vi "SeretBallExercise.vi"(1 "ROUND":dbl) -> ()   [LabVIEW 2013]
uses:
  <vilib>/NXT/Block Support/NXT_OutputPort.ctl
  <vilib>/NXT/Block Support/NXT_InputPort.ctl
  <vilib>/NXT/NXTIO Xnodes/NXTIONodeSubVIs/NXTStopMotors.vi
  <vilib>/NXT/Dual Mode Library/Sensors/EV3_Gyro_Angle.vi
  <vilib>/NXT/Dual Mode Library/Sensors/EV3_Gyro_Reset.vi
  <vilib>/NXT/Subs/LVHSConnector.ctl
  <vilib>/NXT/NXTIO Xnodes/AddressXNode/NXTIOAddress.xnode
  <vilib>/NXT/NXTIO Xnodes/NXTIOXNode/NXTIO.xnode
  <vilib>/NXT/LegoClasses/BrickReference/BrickReference.lvclass
panel:
  out "Numeric":dbl
  out "isBlack2":bool
  out "Degrees 2":sgl
  in  "stop 2":bool
  in  "stop":bool
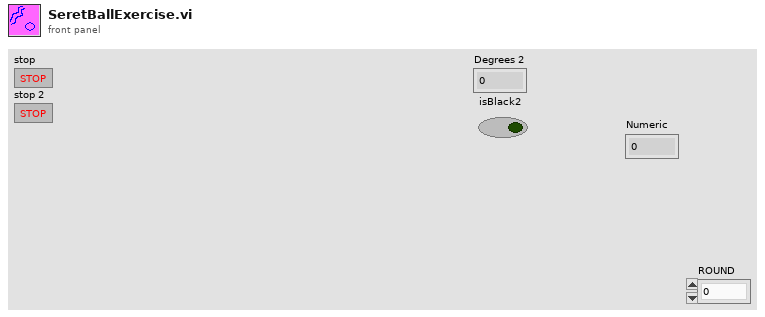
[diagram p1: front panel]
types:
  T1 = typedef "NXT_OutputPort.ctl" = u8
  T2 = typedef "NXT_InputPort.ctl" = u32
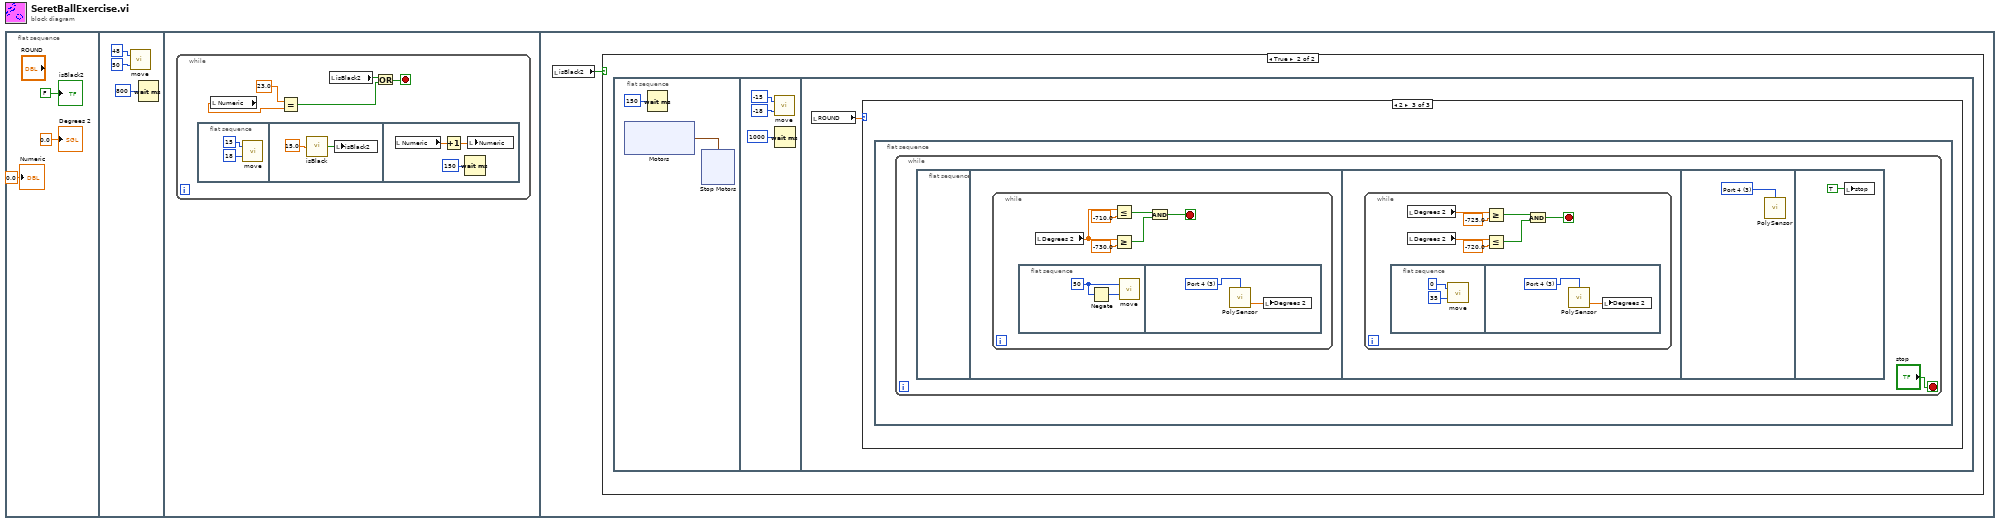
[diagram p0: block diagram]
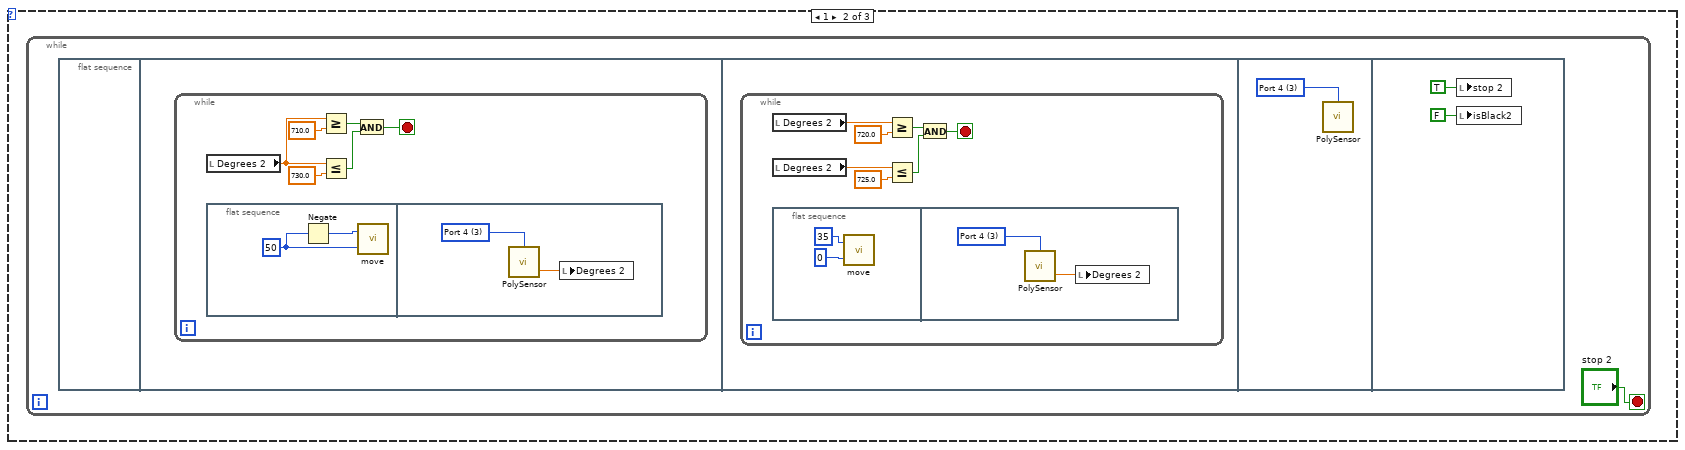
[diagram p4: hidden frame]
diagram:
  n1 = flat-sequence {
    frame #0 {
      "Degrees 2" <- sgl 0.0 ("Degrees 2")
      "isBlack2" <- FALSE ("isBlack2")
      "Numeric" <- 0.0 ("Numeric")
    }
    frame #1 {
      n2 = call "move.vi"("speedLeft"=i8 50, "speedRight"=i8 48) -> ()  [unwired: 1 in]
      n3 = Wait (ms)(milliseconds to wait=u32 800) -> ()  [unwired: 1 out]
    }
    frame #2 {
      n4 = while {
        stop <- w10 stop-if-true
        n5 = flat-sequence {
          frame #0 {
            n6 = call "move.vi"("speedLeft"=i8 18, "speedRight"=i8 15) -> ()  [unwired: 1 in]
          }
          frame #1 {
            n7 = call "isBlack.vi"("BlackBOND"=15.0) -> ("isBlack"=w14:bool)
            n8 = local write "isBlack2"(w14) -> ()
          }
          frame #2 {
            n9 = local read "Numeric"() -> (w17:dbl)
            n10 = Increment(x=w17) -> (x+1=w18:dbl)
            n11 = Wait (ms)(milliseconds to wait=u32 150) -> ()  [unwired: 1 out]
            n12 = local write "Numeric"(w18) -> ()
          }
        }
        n13 = local read "Numeric"() -> (w9:dbl)
        n14 = Equal?(x=23.0, y=w9) -> (x = y?=w7:bool)
        n15 = local read "isBlack2"() -> (w11:bool)
        n16 = Or(x=w11, y=w7) -> (x .or. y?=w10:bool)
      }
    }
    frame #3 {
      n17 = local read "isBlack2"() -> (w19:bool)
      n18 = case shown="True" w19 {
        frame False {
        }
        frame True {
          n19 = flat-sequence {
            frame #0 {
              n20 = xnode "Motors"() -> ("Motor"=w21:cluster{"Port":T1, "Port":T1})
              n21 = Wait (ms)(milliseconds to wait=u32 150) -> ()  [unwired: 1 out]
              n22 = xnode "Stop Motors"("Motors"=w21) -> ()  [unwired: 1 in, 1 out]
            }
            frame #1 {
              n23 = call "move.vi"("speedLeft"=i8 -18, "speedRight"=i8 -15) -> ()  [unwired: 1 in]
              n24 = Wait (ms)(milliseconds to wait=u32 1000) -> ()  [unwired: 1 out]
            }
            frame #2 {
              n25 = local read "ROUND"() -> (w31:dbl)
              n26 = case shown="2" w31 {
                frame 0, Default {
                }
                frame 1 {
                  n27 = while {
                    stop <- "stop 2" stop-if-true
                    n28 = flat-sequence {
                      frame #0 {
                      }
                      frame #1 {
                        n29 = while {
                          stop <- w34 stop-if-true
                          n30 = local read "Degrees 2"() -> (w38:sgl)
                          n31 = flat-sequence {
                            frame #0 {
                              w40 = i8 50 ("speedLeft")
                              n32 = Negate(x=w40) -> (-x=w39:i8)
                              n33 = call "move.vi"("speedLeft"=w40, "speedRight"=w39) -> ()  [unwired: 1 in]
                            }
                            frame #1 {
                              w42 = T2 3 items=["Port 1", "Port 2", "Port 3", "Port 4"] ("Port (Port 1)")
                              n34 = call-poly <vilib>:"PolySensor.vi"("Port (Port 1)"=w42) -> ("Degrees"=w41:sgl)  [unwired: 2 in, 1 out]
                              n35 = local write "Degrees 2"(w41) -> ()
                            }
                          }
                          n36 = Greater Or Equal?(x=w38, y=sgl 710.0) -> (x >= y?=w36:bool)
                          n37 = Less Or Equal?(x=w38, y=730.0) -> (x <= y?=w35:bool)
                          n38 = And(x=w36, y=w35) -> (x .and. y?=w34:bool)
                        }
                      }
                      frame #2 {
                        n39 = while {
                          stop <- w44 stop-if-true
                          n40 = local read "Degrees 2"() -> (w48:sgl)
                          n41 = local read "Degrees 2"() -> (w47:sgl)
                          n42 = flat-sequence {
                            frame #0 {
                              n43 = call "move.vi"("speedLeft"=i8 0, "speedRight"=i8 35) -> ()  [unwired: 1 in]
                            }
                            frame #1 {
                              w52 = T2 3 items=["Port 1", "Port 2", "Port 3", "Port 4"] ("Port (Port 1)")
                              n44 = call-poly <vilib>:"PolySensor.vi"("Port (Port 1)"=w52) -> ("Degrees"=w53:sgl)  [unwired: 2 in, 1 out]
                              n45 = local write "Degrees 2"(w53) -> ()
                            }
                          }
                          n46 = Greater Or Equal?(x=w48, y=sgl 720.0) -> (x >= y?=w45:bool)
                          n47 = Less Or Equal?(x=w47, y=sgl 725.0) -> (x <= y?=w43:bool)
                          n48 = And(x=w45, y=w43) -> (x .and. y?=w44:bool)
                        }
                      }
                      frame #3 {
                        w54 = T2 3 items=["Port 1", "Port 2", "Port 3", "Port 4"] ("Port (Port 1)")
                        n49 = call-poly <vilib>:"PolySensor.vi"("Port (Port 1)"=w54) -> ()  [unwired: 3 in, 1 out]
                      }
                      frame #4 {
                        n50 = local write "stop 2"(TRUE ("stop 2")) -> ()
                        n51 = local write "isBlack2"(FALSE ("isBlack2")) -> ()
                      }
                    }
                  }
                }
                frame 2 {
                  n52 = flat-sequence {
                    frame #0 {
                      n53 = while {
                        stop <- "stop" stop-if-true
                        n54 = flat-sequence {
                          frame #0 {
                          }
                          frame #1 {
                            n55 = while {
                              stop <- w59 stop-if-true
                              n56 = flat-sequence {
                                frame #0 {
                                w65 = i8 50 ("speedRight")
                                n57 = Negate(x=w65) -> (-x=w64:i8)
                                n58 = call "move.vi"("speedLeft"=w64, "speedRight"=w65) -> ()  [unwired: 1 in]
                                }
                                frame #1 {
                                w67 = T2 3 items=["Port 1", "Port 2", "Port 3", "Port 4"] ("Port (Port 1)")
                                n59 = call-poly <vilib>:"PolySensor.vi"("Port (Port 1)"=w67) -> ("Degrees"=w66:sgl)  [unwired: 2 in, 1 out]
                                n60 = local write "Degrees 2"(w66) -> ()
                                }
                              }
                              n61 = local read "Degrees 2"() -> (w58:sgl)
                              n62 = Less Or Equal?(x=w58, y=sgl -710.0) -> (x <= y?=w63:bool)
                              n63 = Greater Or Equal?(x=w58, y=-730.0) -> (x >= y?=w62:bool)
                              n64 = And(x=w63, y=w62) -> (x .and. y?=w59:bool)
                            }
                          }
                          frame #2 {
                            n65 = while {
                              stop <- w69 stop-if-true
                              n66 = flat-sequence {
                                frame #0 {
                                n67 = call "move.vi"("speedLeft"=i8 35, "speedRight"=i8 0) -> ()  [unwired: 1 in]
                                }
                                frame #1 {
                                w77 = T2 3 items=["Port 1", "Port 2", "Port 3", "Port 4"] ("Port (Port 1)")
                                n68 = call-poly <vilib>:"PolySensor.vi"("Port (Port 1)"=w77) -> ("Degrees"=w78:sgl)  [unwired: 2 in, 1 out]
                                n69 = local write "Degrees 2"(w78) -> ()
                                }
                              }
                              n70 = local read "Degrees 2"() -> (w73:sgl)
                              n71 = local read "Degrees 2"() -> (w72:sgl)
                              n72 = Greater Or Equal?(x=w73, y=sgl -725.0) -> (x >= y?=w70:bool)
                              n73 = Less Or Equal?(x=w72, y=sgl -720.0) -> (x <= y?=w68:bool)
                              n74 = And(x=w70, y=w68) -> (x .and. y?=w69:bool)
                            }
                          }
                          frame #3 {
                            w79 = T2 3 items=["Port 1", "Port 2", "Port 3", "Port 4"] ("Port (Port 1)")
                            n75 = call-poly <vilib>:"PolySensor.vi"("Port (Port 1)"=w79) -> ()  [unwired: 3 in, 1 out]
                          }
                          frame #4 {
                            n76 = local write "stop"(TRUE ("stop")) -> ()
                          }
                        }
                      }
                    }
                  }
                }
              }
            }
          }
        }
      }
    }
  }
